vi "Do.vi"(8 "error in (no error)":errorcluster, 9 "Events":refnum<class "Events.lvclass">, 10 "Message Loop Data in":T1, 11 "ResultHanlder JSON":refnum<class "ResultHandler JSON.lvclass">) -> (0 "error out":errorcluster, 2 "Message Loop Data out":T1, 3 "ResultHandler JSOn":refnum<class "ResultHandler JSON.lvclass">)   [LabVIEW 2020, in "wamplv.lvlib" / "ResultHandler JSON.lvclass"]
uses:
  ResultHandler JSON.lvclass
  ResultHandler JSON.lvclass/ResultHandler JSON.ctl
  WAMP Client/API/TypeDefs/RESULT payload (JSON).ctl
  WAMP Client/WAMP Client.lvclass
  WAMP Client/API/TypeDefs/Error or abort detail (JSON).ctl
  wamplv.lvlib
  Events/JsonEvents/JsonEvents.lvclass
  Call/CallRequest (JSON)/CallRequest (JSON).lvclass
  <vilib>/ErrorRing/Error Ring.xnode
  <vilib>/Utility/error.llb/Error Cluster From Error Code.vi
  Error/ErrorHandler JSON/ErrorHandler JSON.lvclass
  a82d7d77-94e0-4436-8633-1ae4a86dbb60.vi
  SerialisedMessages/JSONMessage/WampMessage JSON.lvclass
  Utils/Utils.lvclass
  C:/local/wamplv/Private/SerialisedMessages/JSONMessage/WampMessage JSON.lvclass
  C:/local/wamplv/Private/SerialisedMessages/IWampMessage/IWampMessage.lvclass
  WAMP Client/Private/TypeDef/Publish Requests Map.ctl
  WAMP Client/Private/TypeDef/Endpoint Data.ctl
  Call/ICallRequest/ICallRequest.lvclass
  WAMP Client/Private/TypeDef/CALL Request Map.ctl
  WAMP Client/Private/TypeDef/SUBSCRIBE Requests Map.ctl
  WAMP Client/Private/TypeDef/Subscriptions Map.ctl
  WAMP Client/Private/TypeDef/Unsubscribe Requests Map.ctl
  WAMP Client/Private/TypeDef/Unregister requests map.ctl
  WAMP Client/Private/TypeDef/Message Loop Data.ctl
  Events/EventsParent/Events.lvclass
  Subscribe/ISubscribe/ISubscribe.lvclass
  Publish/IPublish/IPublish.lvclass
  Message loop classes/Subscription details/SubscriptionDetailsParent/SubscriptionDetailsParent.lvclass
  Unsubscribe/IUnsubscribe/IUnsubscribe.lvclass
  Register/IRegister/IRegister.lvclass
  Unregister/IUnregister/IUnregister.lvclass
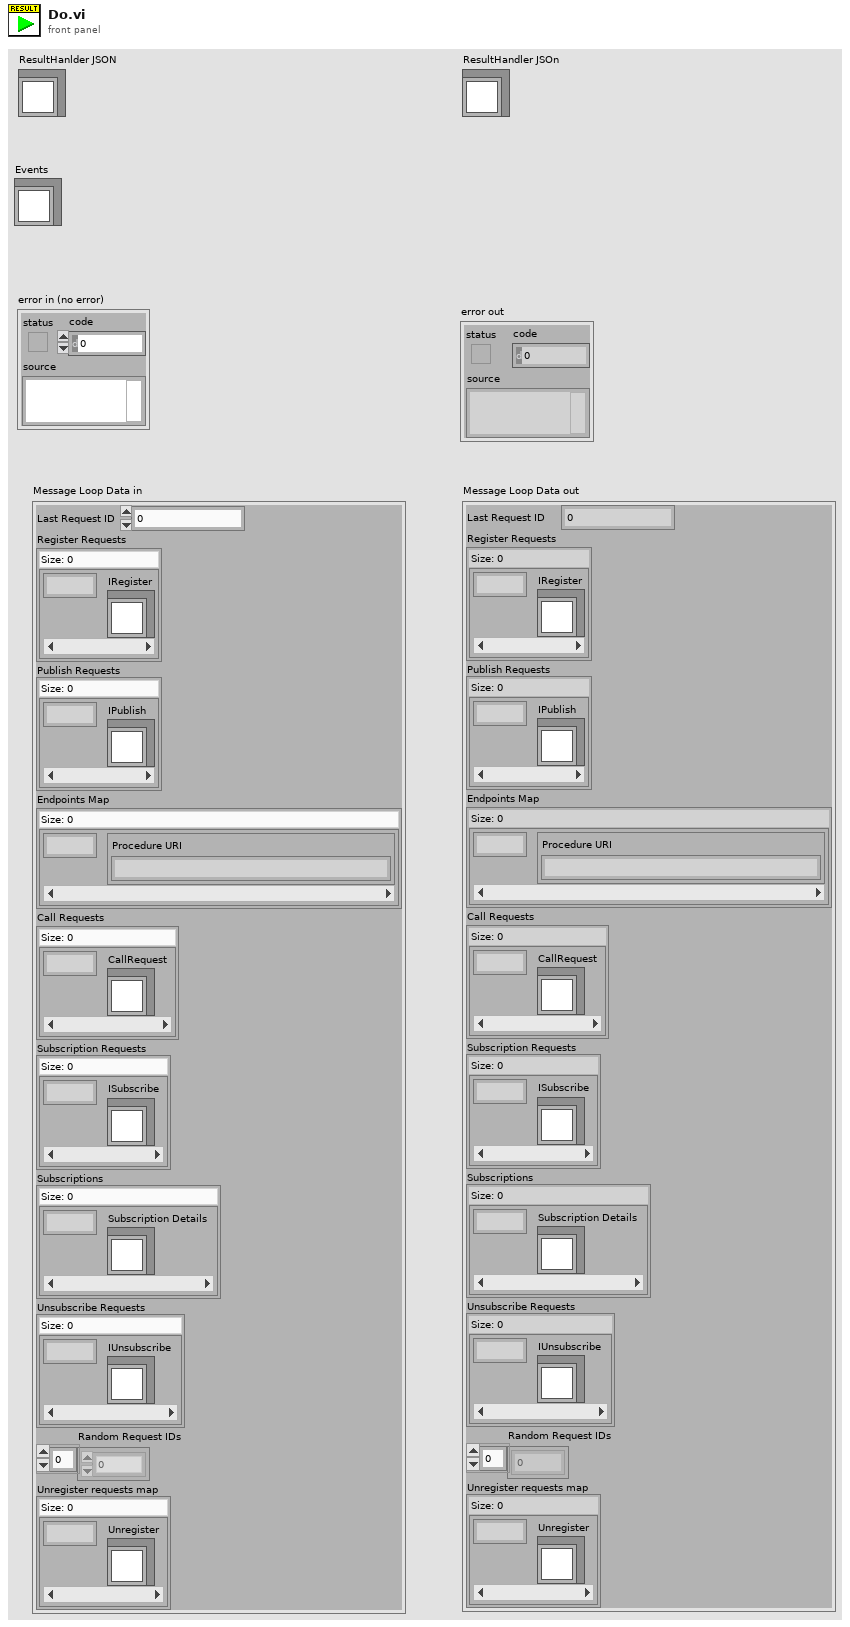
[diagram p1: front panel]
types:
  T1 = typedef "wamplv.lvlib/Message Loop Data.ctl" = cluster{"Last Request ID":u64, "Register Requests":map{u64, refnum<class "IRegister.lvclass">}, "Publish Requests":T2, "Endpoints Map":map{u64, T3}, "Call Requests":T4, "Subscription Requests":T5, "Subscriptions":T6, "Unsubscribe Requests":T7, "Random Request IDs":u64[], "Unregister requests map":T8}
  T2 = typedef "wamplv.lvlib/Publish Requests Map.ctl" = map{u64, refnum<class "IPublish.lvclass">}
  T3 = typedef "wamplv.lvlib/Endpoint Data.ctl" = cluster{"Procedure URI":string}
  T4 = typedef "wamplv.lvlib/CALL Request Map.ctl" = map{u64, refnum<class "ICallRequest.lvclass">}
  T5 = typedef "wamplv.lvlib/SUBSCRIBE Requests Map.ctl" = map{u64, refnum<class "ISubscribe.lvclass">}
  T6 = typedef "wamplv.lvlib/Subscriptions Map.ctl" = map{u64, refnum<class "SubscriptionDetailsParent.lvclass">}
  T7 = typedef "wamplv.lvlib/Unsubscribe Requests Map.ctl" = map{u64, refnum<class "IUnsubscribe.lvclass">}
  T8 = typedef "wamplv.lvlib/Unregister requests map.ctl" = map{u64, refnum<class "IUnregister.lvclass">}
  T9 = typedef "wamplv.lvlib/WAMP Client.lvclass/RESULT payload (JSON).ctl" = cluster{"Topic":string, "Arguments Payload":string, "ArgumentKw Payload":string, "Details":string, "Error/Abort details (JSON)":T10}
  T10 = typedef "wamplv.lvlib/Error or abort detail (JSON).ctl" = cluster{"Error URI":string, "Error Arguments":string, "Error ArgumentKw":string, "Error Details":string, "Associated LabVIEW Error":errorcluster}
  T11 = typedef "wamplv.lvlib/WAMP Message Codes.ctl" = enum8{"HELLO", "WELCOME", "CHALLENGE", "AUTHENTICATE", "ABORT", "GOODBYE", "ERROR", "PUBLISH", "PUBLISHED", "SUBSCRIBE", "SUBSCRIBED", "UNSUBSCRIBE", "UNSUBSCRIBED", "EVENT", "CALL", "RESULT", "REGISTER", "REGISTERED", "UNREGISTER", "UNREGISTERED", "INVOCATION", "YIELD"}
  T12 = typedef "wamplv.lvlib/Error (JSON).ctl" = cluster{"Request ID":u64, "Message type that caused error":T11, "Error/Abort details (JSON)":T10}
  T13 = typedef "wamplv.lvlib/CALL request (JSON).ctl" = cluster{"Topic URI":string, "Arguments":string, "ArgumentsKw":string, "Options":string, "Call result":refnum<notifier>}
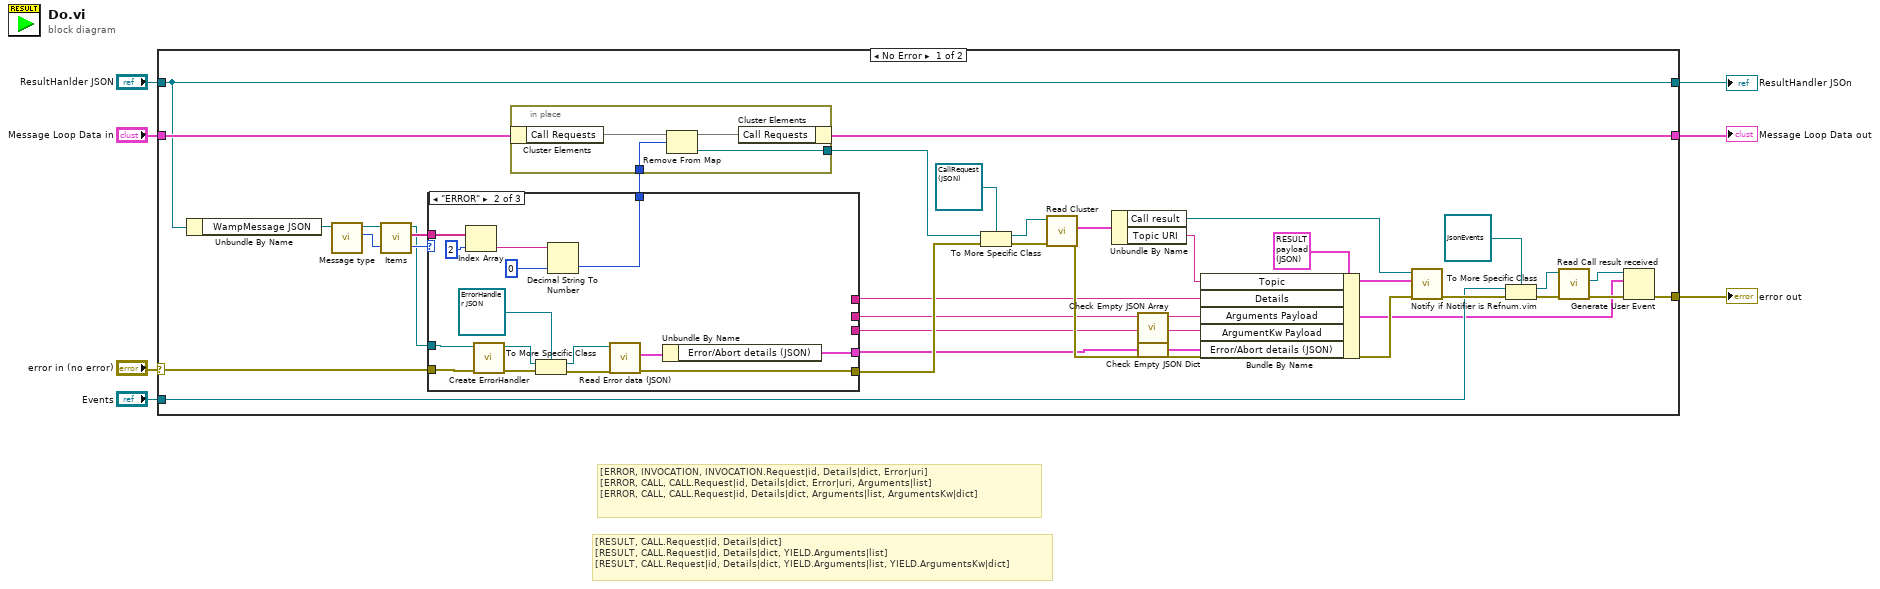
[diagram p0: block diagram]
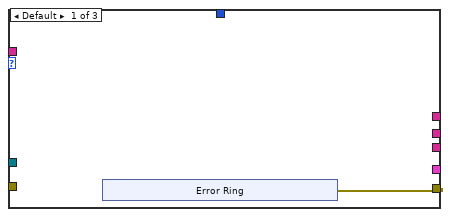
[diagram p2: hidden frame]
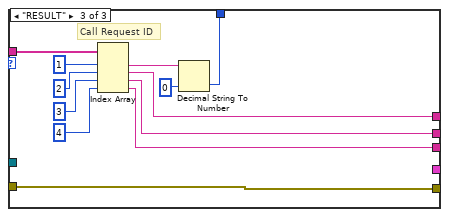
[diagram p3: hidden frame]
diagram:
  # "[RESULT, CALL.Request|id, Details|dict]\n[RESULT, CALL.Request|id, Details|dict, YIELD.Arguments|list]\n[RESULT, CALL.Request|id, Details|dict, YIELD.Arguments|list, YIELD.ArgumentsKw|dict]"
  # "[ERROR, INVOCATION, INVOCATION.Request|id, Details|dict, Error|uri]\n[ERROR, CALL, CALL.Request|id, Details|dict, Error|uri, Arguments|list]\n[ERROR, CALL, CALL.Request|id, Details|dict, Arguments|list, ArgumentsKw|dict]"
  n1 = case shown="No Error" "error in (no error)" {
    selector: "error in (no error)" -> [w16 w80]
    tunnel: "Message Loop Data in" -> [w31 w79]
    tunnel: [w30 w79] -> w6
    tunnel: [w26 w80] -> w5
    tunnel: "Events" -> [w21 _]
    tunnel: "ResultHanlder JSON" -> [w8 w81]
    tunnel: [w8 w81] -> w1
    frame No Error {
      n2 = Unbundle By Name(w8) -> ("WampMessage JSON"=w17:refnum<class "WampMessage JSON.lvclass">)
      n3 = call-dynamic "Message type.vi"("JSONMessage in"=w17) -> ("Message Codes"=w29:T11, "JSONMessage out"=w28:refnum<class "WampMessage JSON.lvclass">)  [unwired: 9 in]
      n4 = call-dynamic "Items.vi"("JSONMessage in"=w28) -> ("<JSON>Elements"=w27:string[], "JSONMessage out"=w18:refnum<class "WampMessage JSON.lvclass">)  [unwired: 9 in]
      n5 = case shown="\"ERROR\"" w29 {
        tunnel: w27 -> [_ w63 w75]
        tunnel: [_ w64 w74] -> w42
        tunnel: [w47 w54 w73] -> w34
        tunnel: [_ _ w67] -> w10
        tunnel: w16 -> [_ w61 w73]
        tunnel: w18 -> [_ w60 _]
        tunnel: [_ w52 _] -> w15
        tunnel: [_ _ w69] -> w14
        tunnel: [_ _ w68] -> w11
        frame Default {
          n6 = xnode "Error Ring"() -> ("error out"=w47:errorcluster)
        }
        frame "ERROR" {
          # "ERROR"
          n7 = Index Array(array=w63, index=2) -> (element=w65:string)
          n8 = call "Create ErrorHandler.vi"("error in (no error)"=w61, "IWampMessage"=w60) -> ("error out"=w59:errorcluster, "IErrorHandler out"=w58:refnum<class "IErrorHandler.lvclass">)  [unwired: 8 in]
          n9 = To More Specific Class(target class=refnum<class "ErrorHandler JSON.lvclass"> refnum ("wamplv.lvlib:ErrorHandler JSON.lvclass"), reference=w58, error in=w59) -> (specific class reference=w55:refnum<class "ErrorHandler JSON.lvclass">, error out=w56:errorcluster)
          n10 = Decimal String To Number(string=w65, default (0L)=u64 0 ("default (0 I32)")) -> (number=w64:u64)  [unwired: 1 in, 1 out]
          n11 = call "Read Error data (JSON).vi"("error in (no error)"=w56, "ErrorHandler JSON in"=w55) -> ("error out"=w54:errorcluster, "Error data (JSON)"=w53:T12)  [unwired: 7 in, 1 out]
          n12 = Unbundle By Name(w53) -> ("Error/Abort details (JSON)"=w52:T10)
        }
        frame "RESULT" {
          # "Call Request ID"
          # "RESULT"
          n13 = Index Array(array=w75, index #1=1 ("index"), index #2=2 ("index"), index #3=3 ("index"), index #4=4 ("index")) -> (element #1=w77:string, element #2=w69:string, element #3=w68:string, element #4=w67:string)
          n14 = Decimal String To Number(string=w77, default (0L)=u64 0) -> (number=w74:u64)  [unwired: 1 in, 1 out]
        }
      }
      n15 = in-place "In Place Element Structure" {
        in-place-border: w42 -> [w46]
        in-place-border: [w45] -> w38
        n16 = in-place-cluster #1(w31) -> ("Call Requests"=w44:T4)
        n17 = Remove From Map(10:w46, 11:w44) -> (1:w45:refnum<class "ICallRequest.lvclass">, 3:w43:T4)  [unwired: 1 out]
        n18 = in-place-cluster #1("Call Requests"=w43) -> (w30:T1)
      }
      n19 = To More Specific Class(target class=refnum<class "CallRequest (JSON).lvclass"> refnum ("wamplv.lvlib:CallRequest (JSON).lvclass"), reference=w38, error in=w34) -> (specific class reference=w35:refnum<class "CallRequest (JSON).lvclass">, error out=w36:errorcluster)
      n20 = call "Read Cluster.vi"("error in (no error)"=w36, "CallRequest (JSON) in"=w35) -> ("error out"=w33:errorcluster, "Cluster"=w32:T13)  [unwired: 7 in, 1 out]
      n21 = Unbundle By Name(w32) -> ("Call result"=w40:refnum<notifier>, "Topic URI"=w39:string)
      n22 = call "Check Empty JSON Array.vi"("JSON in"=w11) -> ("JSON out"=w13:string)  [unwired: 10 in]
      n23 = call "Check Empty JSON Dict.vi"("JSON in"=w10) -> ("JSON out"=w12:string)  [unwired: 10 in]
      n24 = Bundle By Name(cluster=T9 {"Topic"="", "Arguments Payload"="", "ArgumentKw Payload"="", "Details"="[]", "Error/Abort details (JSON)"={"Error URI"="", "Error Arguments"="", "Error ArgumentKw"="", "Error Details"="{}", "Associated LabVIEW Error"={"status"=FALSE, "code"=0, "source"=""}}} ("RESULT Payload"), "Topic"=w39, "Details"=w14, "Arguments Payload"=w13, "ArgumentKw Payload"=w12, "Error/Abort details (JSON)"=w15) -> (w9:T9)
      n25 = call "Notify if Notifier is Refnum.vim"("error in (no error)"=w33, "RESULT Payload"=w9, "Notifier in"=w40) -> ("error out"=w22:errorcluster)  [unwired: 8 in]
      n26 = To More Specific Class(target class=refnum<class "JsonEvents.lvclass"> refnum ("wamplv.lvlib:JsonEvents.lvclass"), reference=w21, error in=w22) -> (specific class reference=w24:refnum<class "JsonEvents.lvclass">, error out=w23:errorcluster)
      n27 = call "Read Call result received .vi"("error in (no error)"=w23, "JsonEvents in"=w24) -> ("error out"=w20:errorcluster, "Call result received"=w19:refnum<user-event>)  [unwired: 7 in, 1 out]
      n28 = Generate User Event(user event=w19, event data cluster=w9, error in=w20) -> (error out=w26:errorcluster)  [unwired: 1 in, 1 out]
    }
    frame Error {
    }
  }
  "error out" <- w5
  "ResultHandler JSOn" <- w1
  "Message Loop Data out" <- w6
